vi "Node - Byte Buffer Read - Runtime.vi"(8 "error in (no error)":errorcluster, 11 "Node Data In":T1) -> (0 "error out":errorcluster, 1 "Channel Data Out":dbl[](array[numeric]), 3 "Node Data Out":T1)   [LabVIEW 2016, in "PXImc Router.lvlib"]
uses:
  PXImc Router.lvlib
  Controls/Node/Node - Config.ctl
  <vilib>/NI Veristand/VeriStand Data/Byte Buffer/Byte Buffer.lvclass
  Controls/Node/Node - PXImc Parameters.ctl
  Controls/Node/Node - Writer Data.ctl
  Controls/Node/Node - Ch Properties.ctl
  Controls/Data Type.ctl
  Controls/Node/Node - Readers Data.ctl
  Controls/Node/Node - Reader Data.ctl
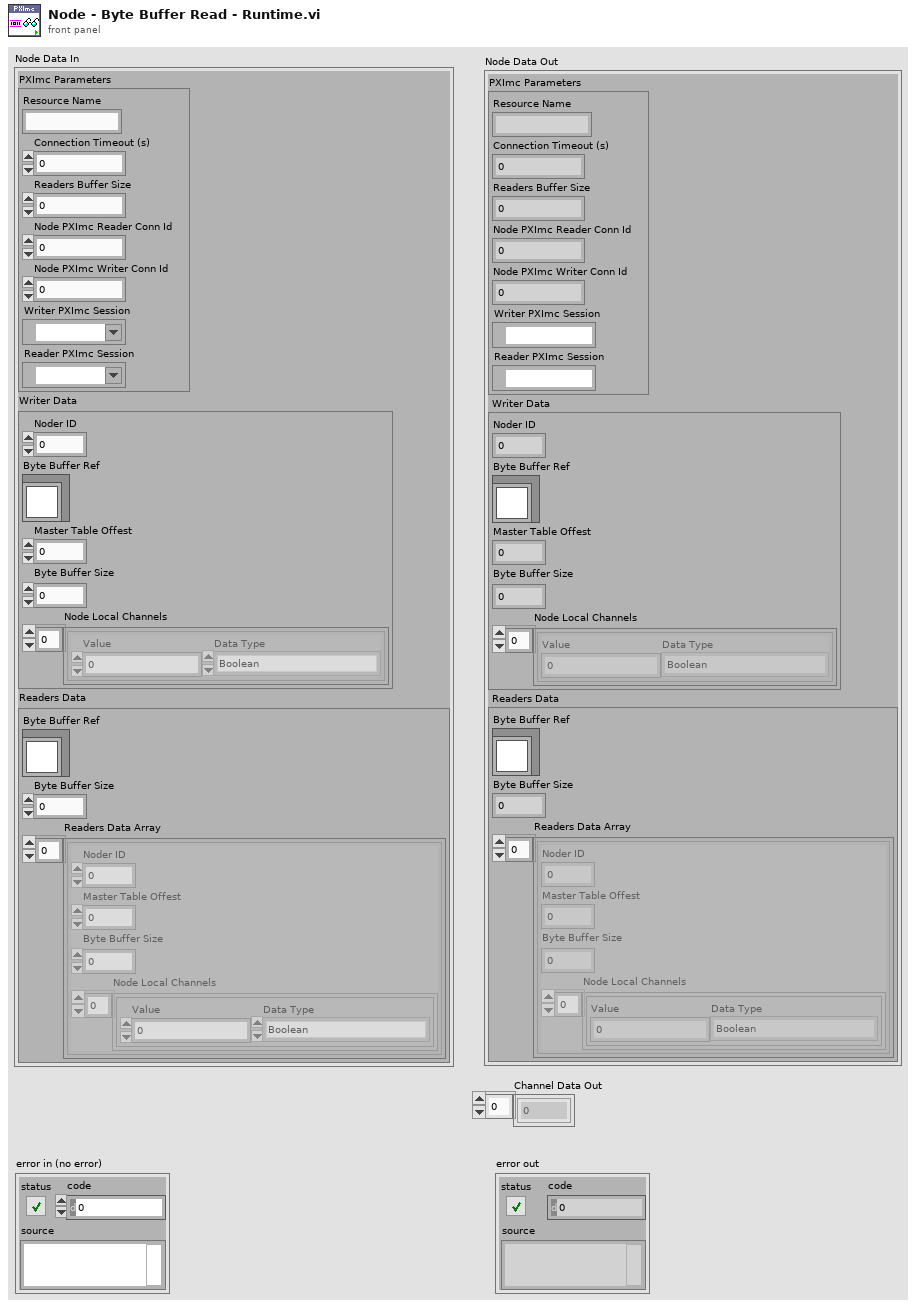
[diagram p1: front panel]
types:
  T1 = typedef "PXImc Router.lvlib/Node - Config.ctl" = cluster{"PXImc Parameters":T2, "Writer Data":T3, "Readers Data":T6}
  T2 = typedef "PXImc Router.lvlib/Node - PXImc Parameters.ctl" = cluster{"Resource Name":string, "Connection Timeout (s)":dbl, "Readers Buffer Size":u64, "Node PXImc Reader Conn Id":u16, "Node PXImc Writer Conn Id":u16, "Writer PXImc Session":refnum<k21>, "Reader PXImc Session":refnum<k21>}
  T3 = typedef "PXImc Router.lvlib/Node - Writer Data.ctl" = cluster{"Noder ID":u32, "Byte Buffer Ref":refnum<class "Byte Buffer.lvclass">, "Master Table Offest":u32, "Byte Buffer Size":u32, "Node Local Channels":T4[]}
  T4 = typedef "PXImc Router.lvlib/Node - Ch Properties.ctl" = cluster{"Value":dbl, "Data Type":T5}
  T5 = typedef "PXImc Router.lvlib/Data Type.ctl" = enum16{"Boolean", "SGL", "DBL", "I8", "I16", "I32", "I64", "U8", "U16", "U32", "U64"}
  T6 = typedef "PXImc Router.lvlib/Node - Readers Data.ctl" = cluster{"Byte Buffer Ref":refnum<class "Byte Buffer.lvclass">, "Byte Buffer Size":u64, "Readers Data Array":T7[]}
  T7 = typedef "PXImc Router.lvlib/Node - Reader Data.ctl" = cluster{"Noder ID":u32, "Master Table Offest":u32, "Byte Buffer Size":u64, "Node Local Channels":T4[]}
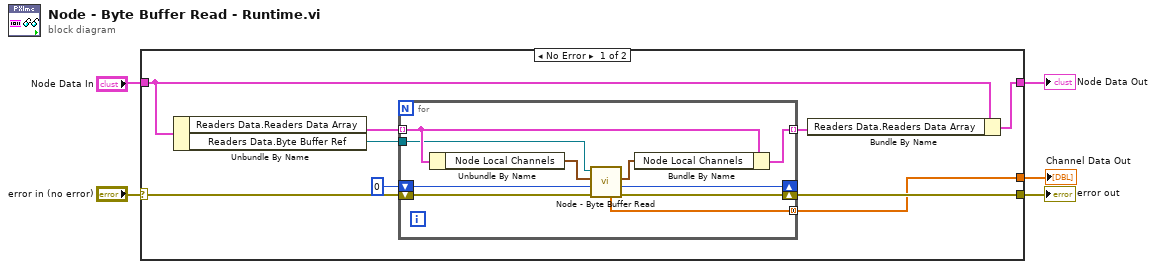
[diagram p0: block diagram]
diagram:
  n1 = case shown="No Error" "error in (no error)" {
    selector: "error in (no error)" -> [w12 w25]
    tunnel: "Node Data In" -> [w14 w26]
    tunnel: [w13 w26] -> w4
    tunnel: [w11 w25] -> w2
    tunnel: [w8 _] -> w1
    frame No Error {
      n2 = Unbundle By Name(w14) -> ("Readers Data.Readers Data Array"=w10:T7[], "Readers Data.Byte Buffer Ref"=w7:refnum<class "Byte Buffer.lvclass">)
      n3 = for {
        shift-right: [w23] -> w11
        shift-left: w12 -> [w24]
        tunnel: w10 -> [w21] mode=indexing
        tunnel: [w20] -> w9 mode=indexing
        tunnel: [w16] -> w8 mode=concatenating
        tunnel: w7 -> [w18]
        shift-right: [w15] -> _
        shift-left: u64 0 ("Buffer Offset In") -> [w17]
        n4 = Unbundle By Name(w21) -> ("Node Local Channels"=w22:T4[])
        n5 = call "Node - Byte Buffer Read.vi"("error in (no error)"=w24, "Buffer Offset In"=w17, "Node Local Channels In"=w22, "Byte Buffer In"=w18) -> ("error out"=w23:errorcluster, "Buffer Offset Out"=w15:u64, "Node Local Channels Out"=w19:T4[], "Channel Data Out"=w16:dbl[])  [unwired: 3 in, 1 out]
        n6 = Bundle By Name(cluster=w21, "Node Local Channels"=w19) -> (w20:T7)
      }
      n7 = Bundle By Name(cluster=w14, "Readers Data.Readers Data Array"=w9) -> (w13:T1)
    }
    frame Error {
    }
  }
  "error out" <- w2
  "Node Data Out" <- w4
  "Channel Data Out" <- w1
